vi "OM_ToLabVIEW.vi"(8 "error in (no error)":errorcluster, 10 "DbRow":variant, 11 "ObjectMap in":refnum<class "ObjectMap.lvclass">) -> (0 "error out":errorcluster, 1 "found":bool, 3 "ObjectMap out":refnum<class "ObjectMap.lvclass">)   [LabVIEW 2020, in "ORM_lib.lvlib" / "ObjectMap.lvclass"]
uses:
  ObjectMap.lvclass
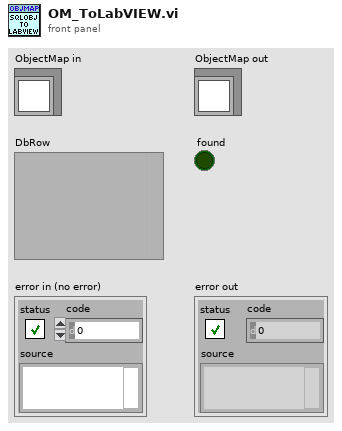
[diagram p1: front panel]
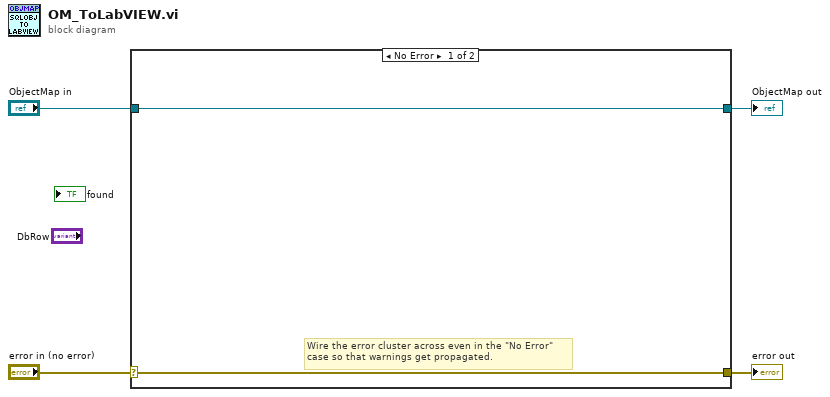
[diagram p0: block diagram]
diagram:
  n1 = case shown="No Error" "error in (no error)" {
    selector: "error in (no error)" -> [w5 w8]
    tunnel: [w5 w8] -> w3
    tunnel: [w6 w7] -> w1
    tunnel: "ObjectMap in" -> [w6 w7]
    frame No Error {
      # "Wire the error cluster across even in the \"No Error\"\ncase so that warnings get propagated."
    }
    frame Error {
    }
  }
  "error out" <- w3
  "ObjectMap out" <- w1
